vi "Find Destination Label.vi"(8 "error in (no error)":errorcluster, 10 "Destination Label":string, 11 "ProjectItem in":refnum<vi>) -> (0 "error IO":errorcluster, 1 "Found":bool, 2 "Destination Name (Tag) out":string, 3 "ProjectItem out":refnum<vi>)   [LabVIEW 2019, in "Project Sync Tools.lvclass"]
uses:
  Project Sync Tools.lvclass
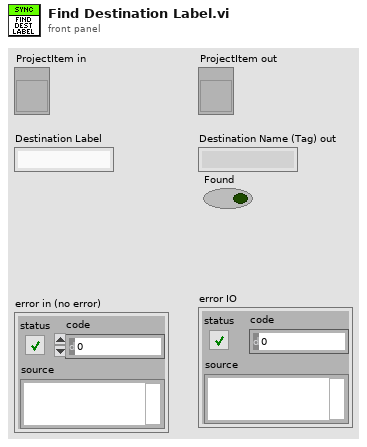
[diagram p1: front panel]
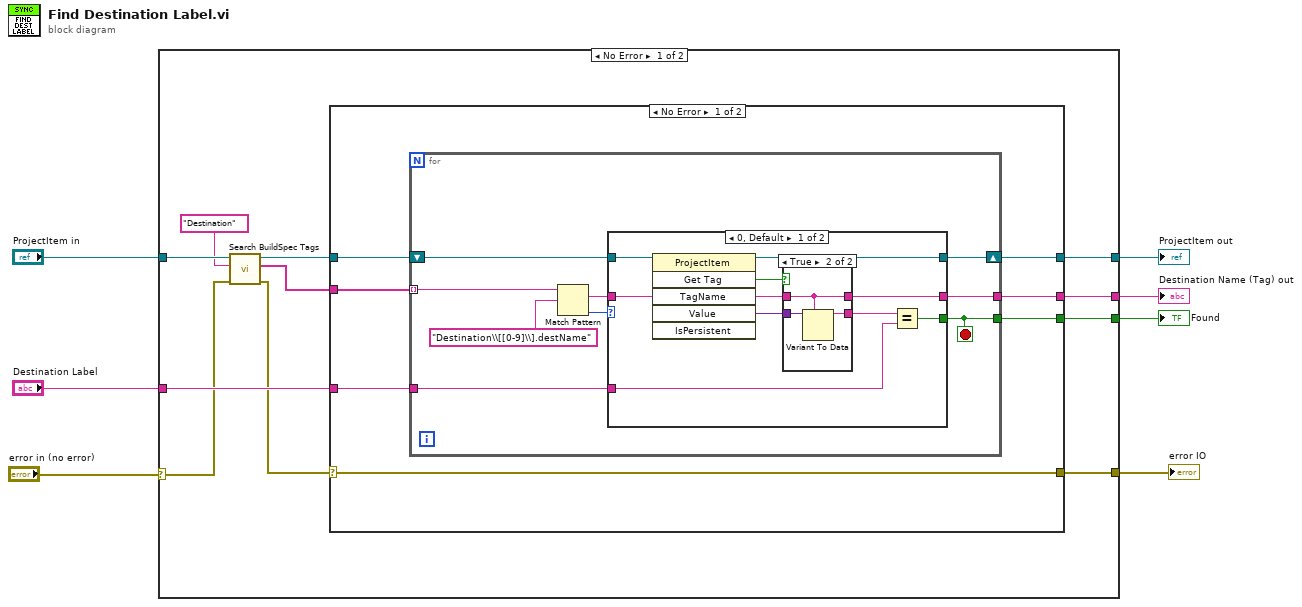
[diagram p0: block diagram]
diagram:
  n1 = case shown="No Error" "error in (no error)" {
    selector: "error in (no error)" -> [w9 w51]
    tunnel: [w18 _] -> w7
    tunnel: [w17 w50] -> w6
    tunnel: [w16 _] -> w5
    tunnel: "Destination Label" -> [w15 _]
    tunnel: "ProjectItem in" -> [w12 w50]
    tunnel: [w8 w51] -> w1
    frame No Error {
      n2 = call "Search BuildSpec Tags.vi"("error in (no error)"=w9, "Regular expression"="Destination", "BuildSpec in"=w12) -> ("error out"=w10:errorcluster, "Tag Names"=w13:string[], "BuildSpec out"=w14:refnum<vi>)  [unwired: 6 in]
      n3 = case shown="No Error" w10 {
        selector: w10 -> [w19 w49]
        tunnel: [w25 _] -> w18
        tunnel: [w24 w48] -> w17
        tunnel: [w23 _] -> w16
        tunnel: w15 -> [w22 _]
        tunnel: w14 -> [w21 w48]
        tunnel: w13 -> [w20 _]
        tunnel: [w19 w49] -> w8
        frame No Error {
          n4 = for {
            tunnel: w20 -> [w31] mode=indexing
            shift-right: [w29] -> w24
            shift-left: w21 -> [w30]
            tunnel: w22 -> [w28]
            tunnel: [w27] -> w23
            tunnel: [w26] -> w25
            stop <- w27 stop-if-true
            n5 = Match Pattern(string=w31, regular expression="Destination\\[[0-9]\\].destName") -> (match substring=w32:string, offset past match=w33:i32)  [unwired: 1 in, 2 out]
            n6 = case shown="0, Default" w33 {
              tunnel: w32 -> [w36 _]
              tunnel: w30 -> [w43 w47]
              tunnel: [w42 w47] -> w29
              tunnel: w28 -> [w38 _]
              tunnel: [w37 _] -> w27
              tunnel: [w35 _] -> w26
              frame 0, Default {
                n7 = invoke class="ProjectItem" method="Get Tag"(reference=w43, "TagName"=w36) -> (reference out=w42:refnum<vi>, "GetTag"=w40:bool, "Value"=w41:variant)  [unwired: 4 in, 3 out]
                n8 = case shown="True" w40 {
                  tunnel: w41 -> [_ w46]
                  tunnel: [_ w45] -> w39
                  tunnel: w36 -> [_ w44]
                  tunnel: [_ w44] -> w35
                  frame False {
                  }
                  frame True {
                    n9 = Variant To Data(type=w44, Variant=w46) -> (data=w45:string)  [unwired: 1 in, 1 out]
                  }
                }
                n10 = Equal?(x=w39, y=w38) -> (x = y?=w37:bool)
              }
              frame -1 {
              }
            }
          }
        }
        frame Error {
        }
      }
    }
    frame Error {
    }
  }
  "Destination Name (Tag) out" <- w7
  "ProjectItem out" <- w6
  "Found" <- w5
  "error IO" <- w1
